vi "Dummy Waypoint Map.vi"() -> ()   [LabVIEW 2012]
panel:
  in  "Obj Simulate":bool
  in  "stop":bool
  in  "Speed":dbl
  in  "Waypoint":i16
  in  "Array":i16[](array[numeric])=[0, 3000, -3000, 3000, -3000, 0]
  out "Motor x out":dbl
  out "Motor y out":dbl
  out "Object Avoid?":bool
  out "XY Graph":cluster{i16[], i16[]}(graph)
  in  "Deg ofset":dbl
  out "Y Pos":i32
  out "X Pos":i32
  in  "Grid Draw":i16=100
  out "Intensity Graph":dbl[][](graph)
  out "Distance left":dbl
  out "Distance right":dbl
  in  "x start":i32=1
  in  "y start":i32=1
  out "X dispacement":i32
  out "Y displacement":i32
  out "Rotation (deg)":dbl
  out "Distance mid":dbl
  out "Finished late":bool
  in  "stop 2":bool
  in  "Boolean":bool
  # "Mapping"
  # "Waypoints"
  # "x"
  # "y"
  # "x start"
  # "y start"
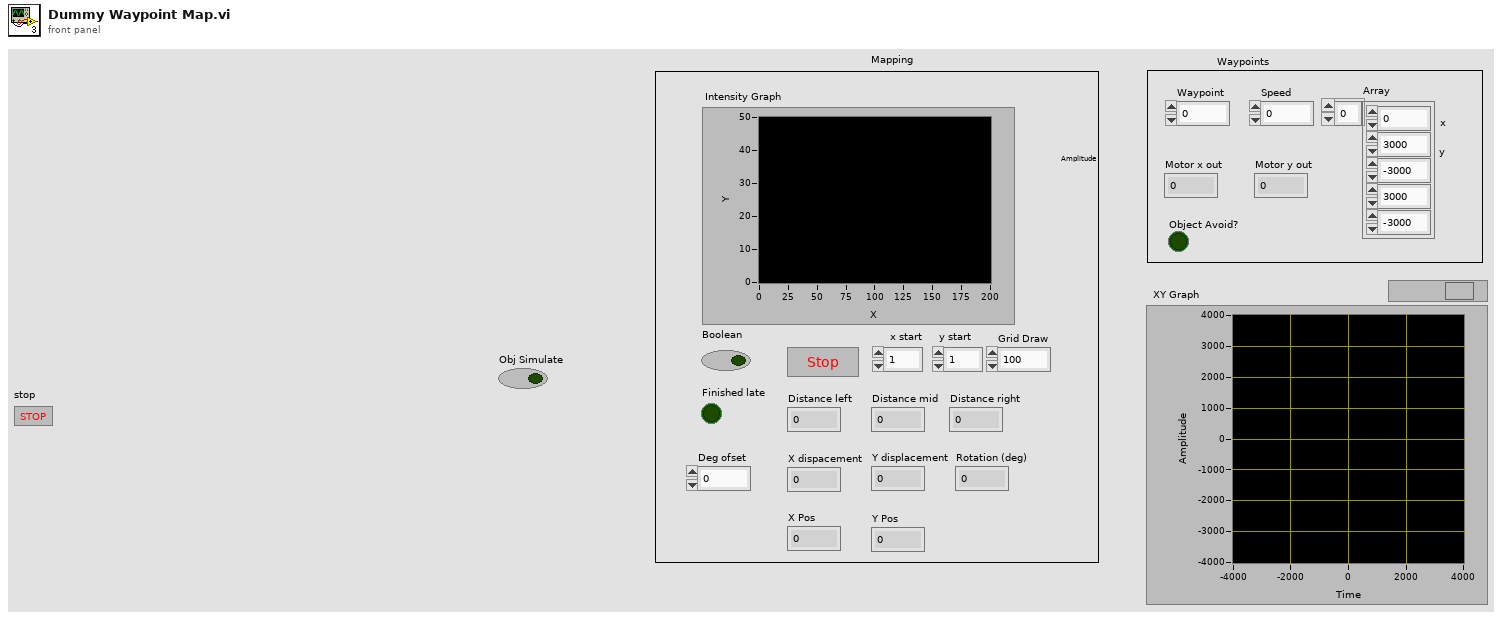
[diagram p1: front panel]
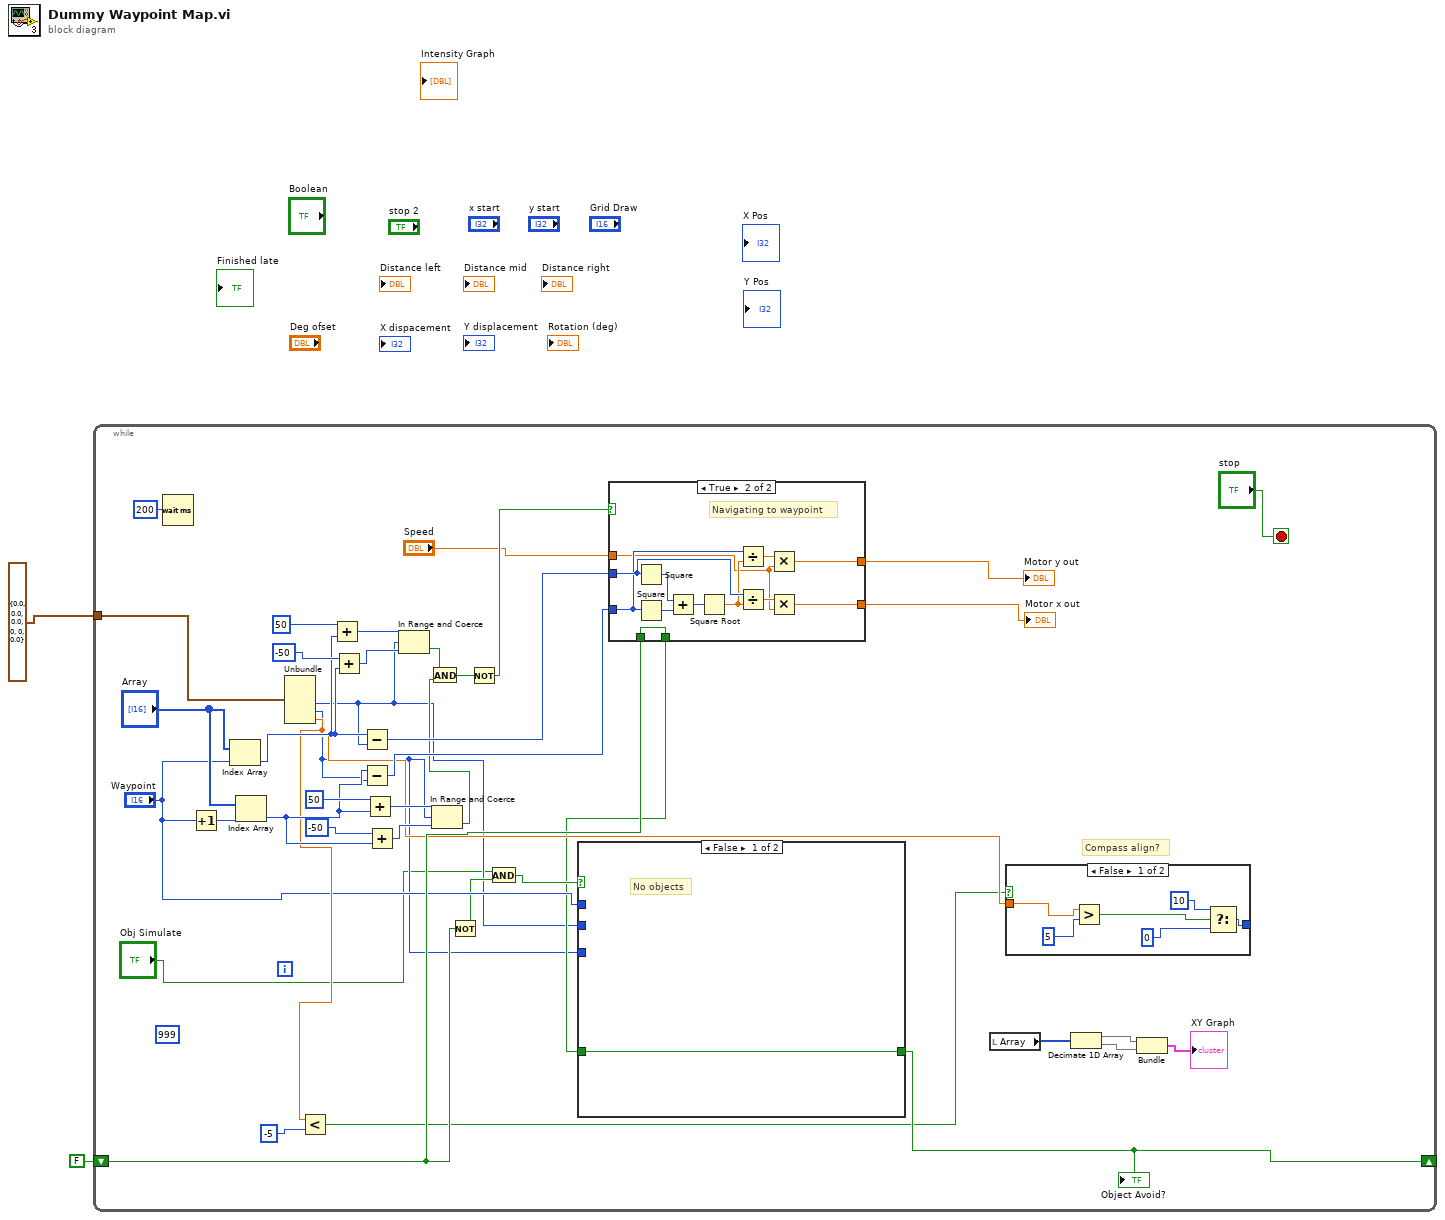
[diagram p0: block diagram]
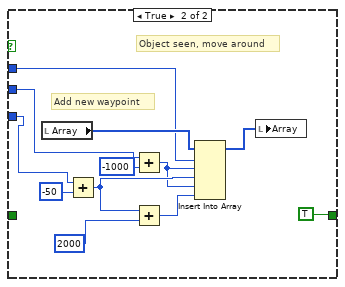
[diagram p2: hidden frame]
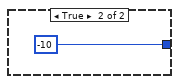
[diagram p3: hidden frame]
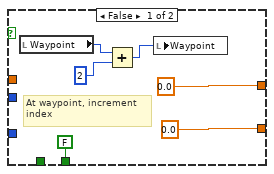
[diagram p4: hidden frame]
diagram:
  n1 = while {
    shift-right: [w38] -> _
    shift-left: FALSE -> [w39]
    tunnel: cluster{dbl, dbl, dbl, i32, i32, dbl} {0.0, 0.0, 0.0, 0, 0, 0.0} ("notification") -> [w4]
    stop <- "stop" stop-if-true
    (unwired) 999
    # "Compass align?"
    n2 = Wait (ms)(milliseconds to wait=200) -> ()  [unwired: 1 out]
    n3 = Increment(x="Waypoint") -> (x+1=w34:i16)
    n4 = Index Array(array="Array", index="Waypoint") -> (element=w27:i16)
    n5 = Index Array(array="Array", index=w34) -> (element=w19:i16)
    n6 = Unbundle(w4) -> (w10:i32, w9:i32, w17:dbl)  [unwired: 3 out]
    n7 = Less?(x=w17, y=-5) -> (x < y?=w15:bool)
    n8 = Add(x=50, y=w27) -> (x+y=w28:i32)
    n9 = Add(x=-50, y=w27) -> (x+y=w30:i32)
    n10 = Subtract(x=w27, y=w10) -> (x-y=w31:i32)
    n11 = Subtract(x=w19, y=w9) -> (x-y=w20:i32)
    n12 = Add(x=50, y=w19) -> (x+y=w22:i32)
    n13 = Add(x=-50, y=w19) -> (x+y=w24:i32)
    n14 = In Range and Coerce(upper limit=w28, x=w10, lower limit=w30) -> (In Range?=w25:bool)  [unwired: 1 out]
    n15 = In Range and Coerce(upper limit=w22, x=w9, lower limit=w24) -> (In Range?=w18:bool)  [unwired: 1 out]
    n16 = And(x=w25, y=w18) -> (x .and. y?=w37:bool)
    n17 = Not(x=w39) -> (.not. x?=w11:bool)
    n18 = Not(x=w37) -> (.not. x?=w36:bool)
    n19 = And(x="Obj Simulate", y=w11) -> (x .and. y?=w13:bool)
    n20 = case shown="True" w36 {
      tunnel: w31 -> [_ w77]
      tunnel: w20 -> [_ w75]
      tunnel: "Speed" -> [_ w72]
      tunnel: [0.0 w71] -> w33
      tunnel: [0.0 w70] -> w40
      tunnel: w39 -> [_ w69]
      tunnel: [FALSE w69] -> w12
      frame False {
        # "At waypoint, increment\nindex"
        n21 = local read "Waypoint"() -> (w66:i16)
        n22 = Add(x=w66, y=2) -> (x+y=w64:i32)
        n23 = local write "Waypoint"(w64) -> ()
      }
      frame True {
        # "Navigating to waypoint"
        n24 = Square(x=w77) -> (x^2=w79:i32)
        n25 = Square(x=w75) -> (x^2=w80:i32)
        n26 = Add(x=w79, y=w80) -> (x+y=w78:i32)
        n27 = Square Root(x=w78) -> (sqrt(x)=w76:dbl)
        n28 = Divide(x=w75, y=w76) -> (x/y=w73:dbl)
        n29 = Divide(x=w77, y=w76) -> (x/y=w74:dbl)
        n30 = Multiply(x=w73, y=w72) -> (x*y=w70:dbl)
        n31 = Multiply(x=w74, y=w72) -> (x*y=w71:dbl)
      }
    }
    "Motor x out" <- w33
    "Motor y out" <- w40
    n32 = case shown="False" w13 {
      tunnel: "Waypoint" -> [_ w54]
      tunnel: w9 -> [_ w52]
      tunnel: w10 -> [_ w50]
      tunnel: w12 -> [w43 _]
      tunnel: [w43 TRUE] -> w38
      frame False {
        # "No objects"
      }
      frame True {
        # "Object seen, move around"
        # "Add new waypoint"
        n33 = local read "Array"() -> (w55:i16[])
        n34 = Add(x=w52, y=-50) -> (x+y=w46:i32)
        n35 = Add(x=w50, y=-1000) -> (x+y=w44:i32)
        n36 = Add(x=w46, y=2000) -> (x+y=w45:i32)
        n37 = Insert Into Array(array=w55, index=w54, new element #1=w44, new element #2=w46, new element #3=w44, new element #4=w45) -> (w49:i16[])
        n38 = local write "Array"(w49) -> ()
      }
    }
    "Object Avoid?" <- w38
    n39 = local read "Array"() -> (w8:i16[])
    n40 = case shown="False" w15 {
      tunnel: w17 -> [w59 _]
      tunnel: [w57 -10] -> _
      frame False {
        n41 = Greater?(x=w59, y=5) -> (0:w60:bool)
        n42 = Select(t=10, s=w60, f=0) -> (s? t:f=w57:i32)
      }
      frame True {
      }
    }
    n43 = Decimate 1D Array(w8) -> (w6:i16[], w5:i16[])
    n44 = Bundle(w6, w5) -> (→"XY Graph":cluster{i16[], i16[]})  [unwired: 1 in]
  }
